vi "Read Arbs.vi"(8 "error in (no error)":errorcluster, 11 "ArbitraryFunction in":refnum<class "ArbitraryFunction.lvclass">) -> (0 "error out":errorcluster, 2 "Arbs":T1[](array[typedef]), 3 "ArbitraryFunction out":refnum<class "ArbitraryFunction.lvclass">)   [LabVIEW 2018, in "Functions.lvlib" / "ArbitraryFunction.lvclass"]
uses:
  ArbitraryFunction.lvclass
  TypeDefs/Arbitrary.ctl
  ArbitraryFunction.lvclass/ArbitraryFunction.ctl
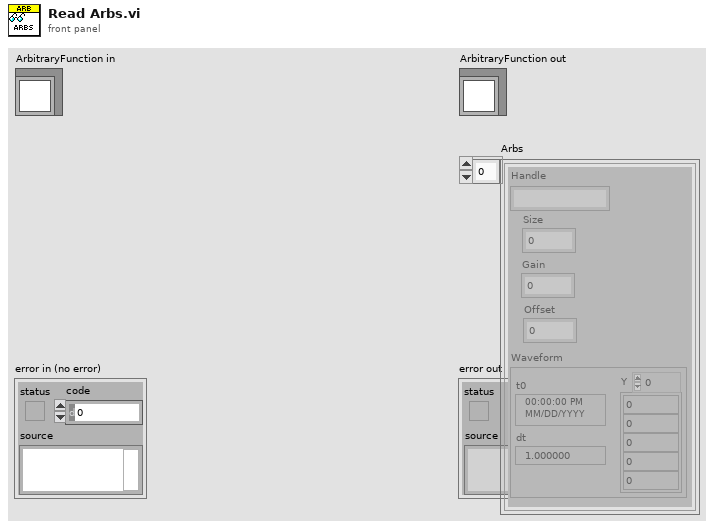
[diagram p1: front panel]
types:
  T1 = typedef "Functions.lvlib/ArbitraryFunction.lvclass/Arbitrary.ctl" = cluster{"Handle":string, "Size":i32, "Gain":dbl, "Offset":dbl, "Waveform":waveform(dbl)}
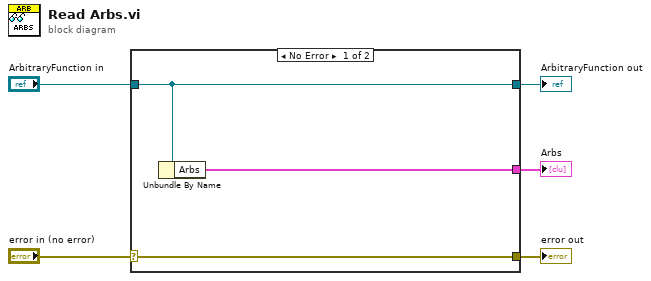
[diagram p0: block diagram]
diagram:
  n1 = case shown="No Error" "error in (no error)" {
    selector: "error in (no error)" -> [w8 w9]
    tunnel: [w8 w9] -> w4
    tunnel: [w7 w10] -> w2
    tunnel: "ArbitraryFunction in" -> [w7 w10]
    tunnel: [w6 _] -> w1
    frame No Error {
      n2 = Unbundle By Name(w7) -> ("Arbs"=w6:T1[])
    }
    frame Error {
    }
  }
  "error out" <- w4
  "ArbitraryFunction out" <- w2
  "Arbs" <- w1
